vi "GE 5565PIORC.Registers.PCIBAR0.Prefetchable.Get.vi"(8 "error in (no error)":errorcluster, 11 "GE 5565PIORC in":refnum<class "GE 5565PIORC.lvclass">) -> (0 "error out":errorcluster, 2 "Prefetchable":bool, 3 "GE 5565PIORC out":refnum<class "GE 5565PIORC.lvclass">)   [LabVIEW 2016, in "GE 5565PIORC.lvclass"]
doc: "Writing a one (1) indicates there are no side effects on reads.\n\n<B>Note:</B> Hardcoded to zero (0)."
uses:
  GE 5565PIORC.lvclass
  GE 5565PIORC.Registers.PCI Configuration.ctl
  GE 5565PIORC.lvclass/GE 5565PIORC.ctl
  GE 5565PIORC.Registers.PCI Configuration.Read (U32).vi
  Bit Manipulation.Get Bit (U32).vi
  GE 5565PIORC.Registers.Read.vi
  GE 5565PIORC.Registers.Read (U32).vi
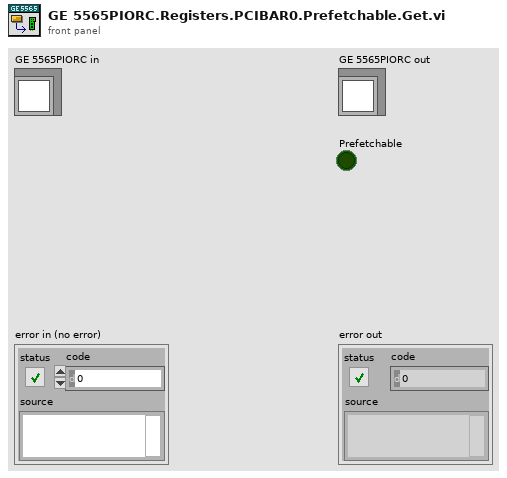
[diagram p1: front panel]
types:
  T1 = typedef "GE 5565PIORC.lvclass/GE 5565PIORC.Registers.PCI Configuration.ctl" = u32
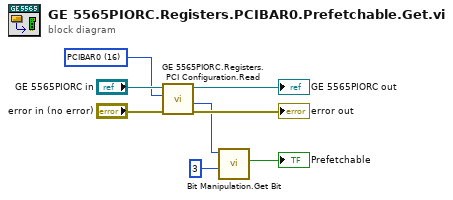
[diagram p0: block diagram]
diagram:
  w3 = T1 16 items=["PCI Configuration ID"=0, "PCI Command"=4, "PCI Status"=6, "PCI Revision ID"=8, "PCI Class Code"=9, "PCI Cache Line Size"=12, "PCI Latency Timer"=13, "PCI Header Type"=14, "PCI Built-in Self Test"=15, "PCIBAR0"=16, "PCIBAR1"=20, "PCIBAR2"=24, "PCIBAR3"=28, "PCIBAR4"=32, "PCIBAR5"=36, "PCI Cardbus CIS Pointer"=40, "PCI Subsystem Vendor ID"=44, "PCI Subsystem ID"=46, "PCI Expansion ROM Base"=48, "Capability Pointer"=52, "PCI Interrupt Line"=60, "PCI Interrupt Pin"=61, "PCI Min_Gnt"=62, "PCI Max_Lat"=63] ("Register")
  n1 = call-poly "GE 5565PIORC.Registers.PCI Configuration.Read.vi"("error in (no error)"="error in (no error)", "Register"=w3, "GE 5565PIORC in"="GE 5565PIORC in") -> ("error out"=→"error out":errorcluster, "Value"=w4:u32, "GE 5565PIORC out"=→"GE 5565PIORC out":refnum<class "GE 5565PIORC.lvclass">)  [unwired: 6 in]
  n2 = call-poly "Bit Manipulation.Get Bit.vi"("bit index"=3, "packed value in"=w4) -> ("bit"=→"Prefetchable":bool)  [unwired: 8 in, 1 out]
